vi "海流计数据拆分.vi"() -> (2 "不再发送":bool, 3 "当前要发送的海流计参数":string[][](array[string]))   [LabVIEW 2016, in "数据传输系统.lvlib"]
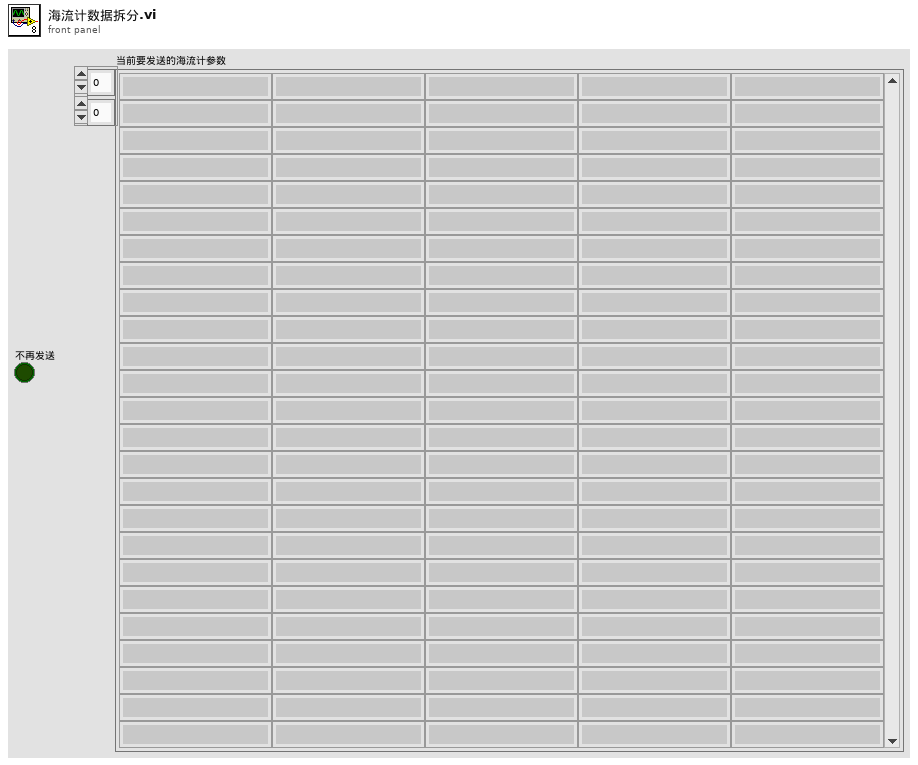
[diagram p1: front panel]
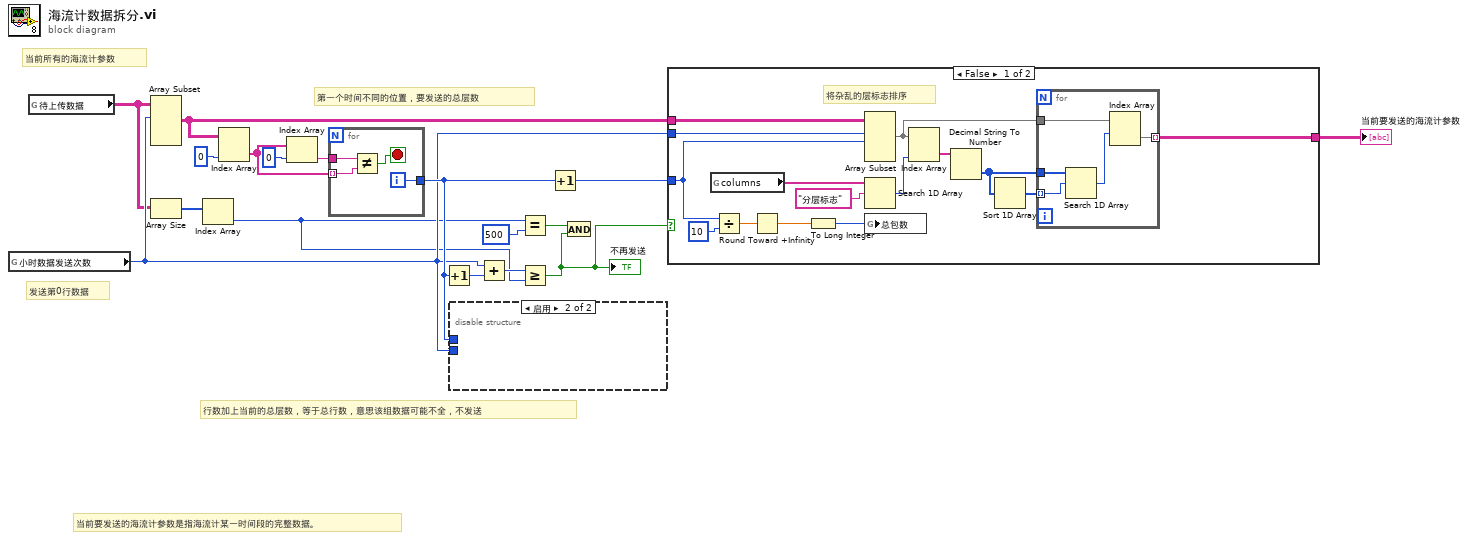
[diagram p0: block diagram]
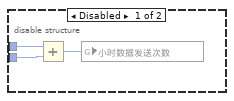
[diagram p2: hidden frame]
diagram:
  # "当前要发送的海流计参数是指海流计某一时间段的完整数据。"
  # "行数加上当前的总层数，等于总行数，意思该组数据可能不全，不发送"
  # "第一个时间不同的位置，要发送的总层数"
  # "发送第0行数据"
  # "当前所有的海流计参数"
  n1 = global read "全局 小时数据发送次数.vi" "小时数据发送次数"() -> (w4:i32)
  n2 = global read "全局 所有参数.vi" "待上传数据"() -> (w1:string[][])
  n3 = Array Subset(array=w1, index (row)=w4) -> (w13:string[][])  [unwired: 3 in]
  n4 = Array Size(array=w1) -> (size(s)=w12:i32[])
  n5 = Index Array(array=w12) -> (element=w3:i32)  [unwired: 1 in]
  n6 = Index Array(array=w13, index (col)=0 ("索引 (行)")) -> (element=w14:string[])  [unwired: 1 in]
  n7 = Index Array(array=w14, index=0 ("索引")) -> (element=w15:string)
  n8 = for {
    tunnel: w15 -> [w18]
    tunnel: [w20] -> w6
    tunnel: w14 -> [w19] mode=indexing
    i -> [w20]
    stop <- w21 stop-if-true
    n9 = Not Equal?(x=w18, y=w19) -> (x != y?=w21:bool)
  }
  n10 = Increment(x=w6) -> (x+1=w9:i32)
  n11 = disable-structure shown="启用" {
    disable-tunnel: w4 -> [w23 _]
    disable-tunnel: w6 -> [w22 _]
    frame Disabled {
      n12 = Add(x=w22, y=w23) -> (x+y=w24:i32)
      n13 = global write "全局 小时数据发送次数.vi" "小时数据发送次数"(w24) -> ()
    }
    frame Enabled {
    }
  }
  n14 = Add(x=w4, y=w9) -> (x+y=w10:i32)
  n15 = Equal?(x=w3, y=500) -> (x = y?=w11:bool)
  n16 = Greater Or Equal?(x=w10, y=w3) -> (x >= y?=w5:bool)
  "不再发送" <- w5
  n17 = Increment(x=w6) -> (x+1=w7:i32)
  n18 = And(x=w11, y=w5) -> ()  [unwired: 1 out]
  n19 = case shown="False" w5 {
    tunnel: w13 -> [w35 _]
    tunnel: w7 -> [w27 _]
    tunnel: [w26 _] -> w2
    tunnel: w4 -> [w25 _]
    frame False {
      # "将杂乱的层标志排序"
      n20 = global read "全局 所有参数.vi" "columns"() -> (w29:string[])
      n21 = Divide(x=w27, y=10) -> (x/y=w38:dbl)
      n22 = Round Toward +Infinity(x=w38) -> (ceil(x): smallest int >= x=w39:dbl)
      n23 = To Long Integer(number=w39) -> (32bit integer=w36:i32)
      n24 = Array Subset(array=w35, index (row)=w25, length (row)=w27) -> (w28:string[][])  [unwired: 2 in]
      n25 = Search 1D Array(1D array=w29, element="分层标志" ("元素")) -> (index of element=w31:i32)  [unwired: 1 in]
      n26 = global write "全局 数据数组大小.vi" "总包数"(w36) -> ()
      n27 = Index Array(array=w28, index (col)=w31) -> (element=w32:string[])  [unwired: 1 in]
      n28 = Decimal String To Number(string=w32) -> (number=w33:i32[])  [unwired: 2 in, 1 out]
      n29 = Sort 1D Array(array=w33) -> (sorted array=w34:i32[])
      n30 = for {
        tunnel: w33 -> [w44]
        tunnel: w34 -> [w43] mode=indexing
        tunnel: w28 -> [w42]
        tunnel: [w40] -> w26 mode=indexing
        n31 = Search 1D Array(1D array=w44, element=w43) -> (index of element=w41:i32)  [unwired: 1 in]
        n32 = Index Array(array=w42, index (row)=w41) -> (element=w40:string[])  [unwired: 1 in]
      }
    }
    frame True {
    }
  }
  "当前要发送的海流计参数" <- w2
